vi "Insert Vi.vi"(8 "error in (no error)":errorcluster caption="错误输入（无错误）", 9 "ViValue":string, 10 "VI*":refnum<vi>, 11 "PanelDataNode 输入":refnum<class "PanelDataNode.lvclass"> caption="DNL_LabVIEW Object in") -> (0 "error out":errorcluster caption="错误输出", 3 "PanelDataNode 输出":refnum<class "PanelDataNode.lvclass"> caption="DNL_LabVIEW Object out")   [LabVIEW 2013, in "PanelDataNode.lvclass"]
uses:
  PanelDataNode.lvclass
  PanelDataNode.lvclass/PanelDataNode.ctl
  PanelLinkNode/PanelLinkNode.lvclass/PanelLinkNode.ctl
  PanelLinkNode/PanelLinkNode.lvclass
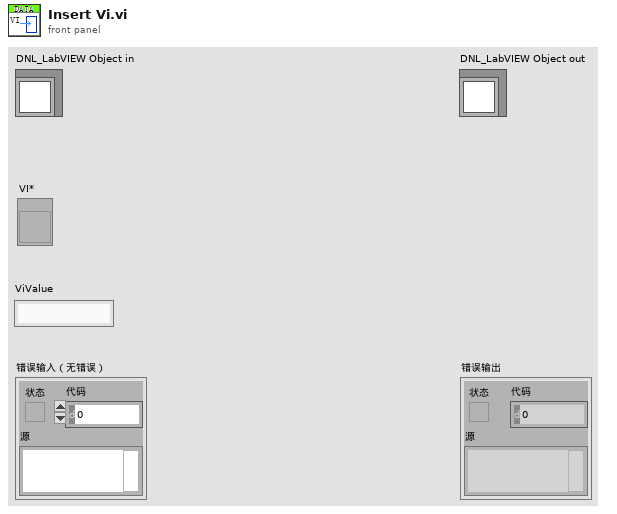
[diagram p1: front panel]
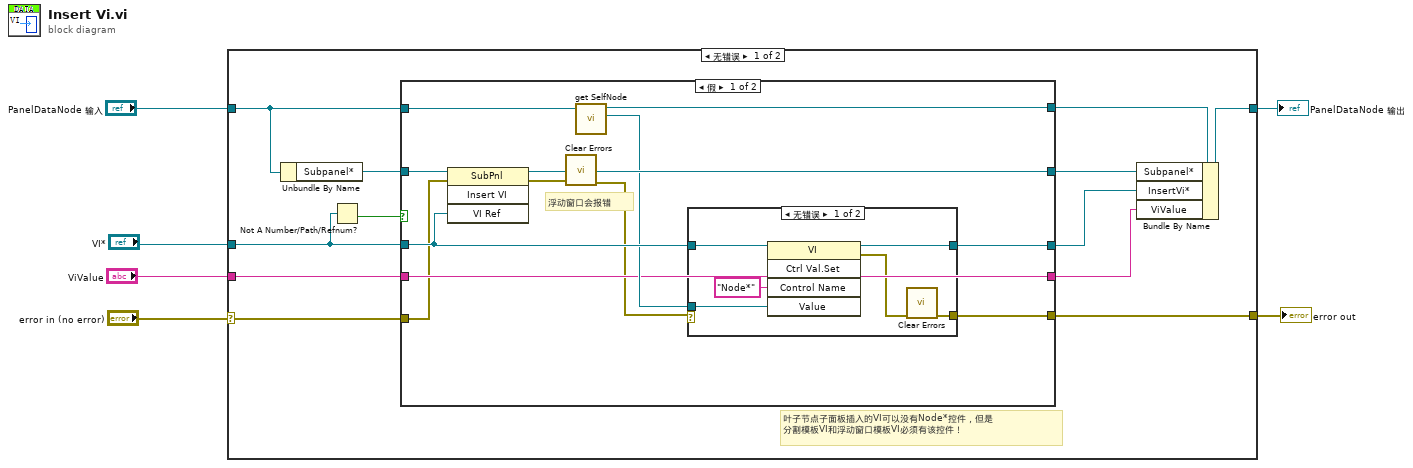
[diagram p0: block diagram]
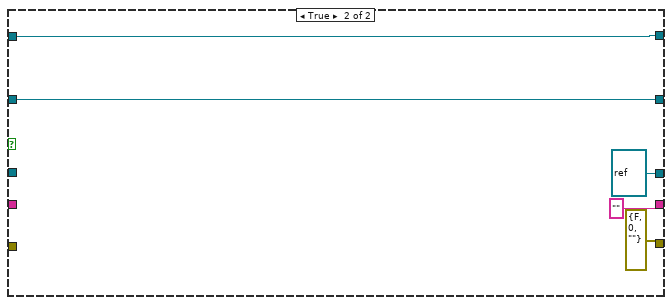
[diagram p3: hidden frame]
diagram:
  n1 = case shown="无错误" "error in (no error)" {
    selector: "error in (no error)" -> [w7 w45]
    tunnel: [w17 w45] -> w5
    tunnel: [w16 w44] -> w3
    tunnel: "PanelDataNode 输入" -> [w12 w44]
    tunnel: "ViValue" -> [w10 _]
    tunnel: "VI*" -> [w8 _]
    frame No Error {
      # "叶子节点子面板插入的VI可以没有Node*控件，但是\n分割模板VI和浮动窗口模板VI必须有该控件！"
      n2 = Unbundle By Name(w12) -> ("Subpanel*"=w18:refnum<vi>)
      n3 = Not A Number/Path/Refnum?(number/path/refnum=w8) -> (NaN/Path/Refnum?=w14:bool)
      n4 = case shown="假" w14 {
        tunnel: w18 -> [w30 w43]
        tunnel: [w25 errorcluster {"status"=FALSE, "code"=0, "source"=""} ("错误输出")] -> w17
        tunnel: [w29 w43] -> w15
        tunnel: w8 -> [w28 _]
        tunnel: [w27 refnum<vi> refnum ("VI*")] -> w13
        tunnel: w12 -> [w26 w42]
        tunnel: [w24 w42] -> w11
        tunnel: w10 -> [w22 _]
        tunnel: [w22 "" ("ViValue")] -> w9
        tunnel: w7 -> [w19 _]
        frame False {
          # "浮动窗口会报错"
          n5 = invoke class="SubPnl" method="Insert VI"(reference=w30, error in=w19, "VI Ref"=w28) -> (reference out=w29:refnum<vi>, error out=w21:errorcluster)  [unwired: 1 in, 2 out]
          n6 = call <vilib>:"Clear Errors.vi"("error in (no error)"=w21) -> ("error out"=w20:errorcluster)  [unwired: 6 in]
          n7 = call "get SelfNode.vi"("PanelLinkNode输入"=w26) -> ("SelfNode*"=w23:refnum<data-value>, "PanelLinkNode输出"=w24:refnum<class "PanelDataNode.lvclass">)  [unwired: 8 in, 1 out]
          n8 = case shown="无错误" w20 {
            selector: w20 -> [_ w38]
            tunnel: w28 -> [w36 w37]
            tunnel: [w35 w37] -> w27
            tunnel: [w32 w38] -> w25
            tunnel: w23 -> [w33 _]
            frame No Error {
              n9 = invoke class="VI" method="Ctrl Val.Set"(reference=w36, "Control Name"="Node*" ("控件名"), "Value"=w33) -> (reference out=w35:refnum<vi>, error out=w31:errorcluster)  [unwired: 2 in, 3 out]
              n10 = call <vilib>:"Clear Errors.vi"("error in (no error)"=w31) -> ("error out"=w32:errorcluster)  [unwired: 6 in]
            }
            frame Error {
            }
          }
        }
        frame True {
        }
      }
      n11 = Bundle By Name(cluster=w11, "Subpanel*"=w15, "InsertVi*"=w13, "ViValue"=w9) -> (w16:refnum<class "PanelDataNode.lvclass">)
    }
    frame Error {
    }
  }
  "error out" <- w5
  "PanelDataNode 输出" <- w3
